vi "comunication break.vi"(8 "错误输入（无错误）":errorcluster, 11 "motor control输入":T1={"System no."=1, "Conn. \nAxes"=[], "当前数值"=[]} {"System no." min=1 step=1}) -> (0 "错误输出":errorcluster)   [LabVIEW 2017]
doc: "本VI是一个因为常用但是老要解绑很麻烦，所以提取出来的一个VI，其作用就是检查仪器时候通讯，如果通讯就断开通讯，为下次连接做准备。"
uses:
  motor control.ctl
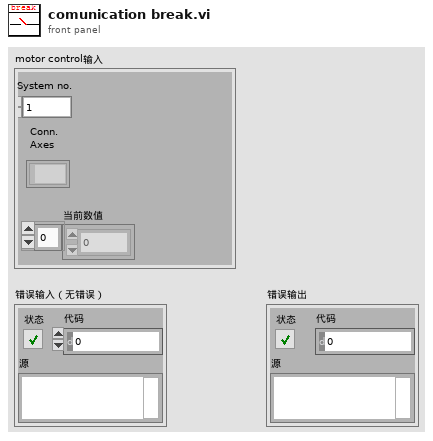
[diagram p1: front panel]
types:
  T1 = typedef "motor control.ctl" = cluster{"System no.":i32, "Conn. \nAxes":string[], "当前数值":dbl[]}
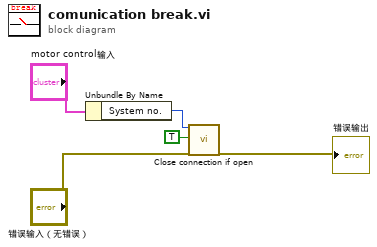
[diagram p0: block diagram]
diagram:
  n1 = Unbundle By Name("motor control输入") -> ("System no."=w2:i32)
  n2 = call "Close connection if open.vi"("System no."=w2, "Close DaisyChain"=TRUE, "error in"="错误输入（无错误）") -> ("error out"=→"错误输出":errorcluster)  [unwired: 15 in, 1 out]
